vi "GetEvents.vi"(8 "Error In":errorcluster, 11 "object in":refnum<class "WebView.JSONEditor.lvclass">) -> (0 "Error Out":errorcluster, 2 "Events":T1, 3 "object out":refnum<class "WebView.JSONEditor.lvclass">)   [LabVIEW 2024, in "WebView.JSONEditor.lvclass"]
uses:
  WebView.JSONEditor.lvclass
  private/JSONEditor Events.ctl
  private/JSON Updated Event Data--cluster.ctl
  private/Seleced Node Path Event Data--string.ctl
  WebView.JSONEditor.lvclass/WebView.JSONEditor.ctl
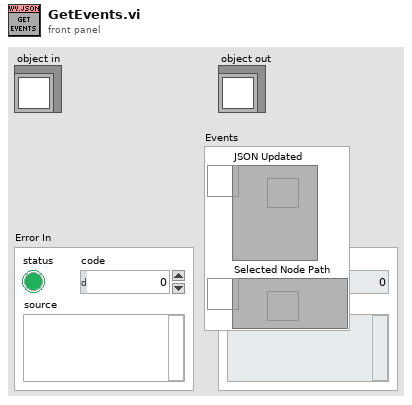
[diagram p1: front panel]
types:
  T1 = typedef "WebView.JSONEditor.lvclass/JSONEditor Events.ctl" = cluster{"JSON Updated":refnum<user-event>, "Selected Node Path":refnum<user-event>}
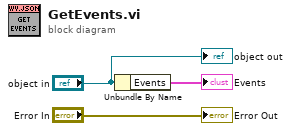
[diagram p0: block diagram]
diagram:
  n1 = Unbundle By Name("object in") -> ("Events"=→"Events":T1)
  "Error Out" <- "Error In"
  "object out" <- "object in"
